vi "RequestFIFO.vi"   [LabVIEW 2018]
uses:
  <vilib>/rvi/Emulation/niFpgaGetClockAttributes.vi
  <vilib>/rvi/Emulation/niFpgaSctlEmulationGetInTimedLoop.vi
  <vilib>/rvi/Emulation/niFpgaEmulationReportErrorSimple.vi
  <vilib>/rvi/interface/RandomDataEmulation/niFpgaRandomDataHandleErrors.vi
  <vilib>/rvi/Emulation/niFpgaEmulationIsFPGAContextNoSignature.vi
  <vilib>/rvi/errors/niFpgaSetErrorForExecOnDevCompSimple.vi
  <vilib>/rvi/eio/common/nirviEmuReportErrorAndStop.vi
  <vilib>/rvi/DataTransferAndStorage/Container/Common/niFpgaContainerGetUniqueNameForEmu.vi
  <vilib>/rvi/FIFO/Fifo_Resource/nirvififoEmulationSetSize.vi
  <vilib>/rvi/FIFO/Fifo_Resource/nirviFifoEmulationQueueMgr.vi
  <instcachedir>/0/nirviFifoEmulationQueueMgr_E5CAEC123FF24DC58D834DCA3CDAA9B5.lvgen/nirviFifoEmulationQueueMgr_E5CAEC123FF24DC58D834DCA3CDAA9B5_032.vi
  <vilib>/Utility/error.llb/Clear Errors.vi
  <vilib>/rvi/FIFO/Fifo_Resource/nirvififoEmulationCreateLock.vi
  <vilib>/rvi/Emulation/niFpgaProcessEmulError.vi
  <vilib>/rvi/FIFO/Fifo_Resource/nirvififoEmulationObtainLock.vi
  <vilib>/rvi/FIFO/Fifo_Resource/nirvififoEmulationReleaseLock.vi
  <vilib>/rvi/occurrence/nirviWaitOnOccurrenceBase.vi
  <vilib>/rvi/errors/nirviReportUnexpectedCaseInternalError.vi
  <vilib>/rvi/errors/nirviReportUnexpectedCaseInternalError (U32).vi
  <vilib>/rvi/eio/common/nirviEmuTemplateMethod_errors.vi
  <vilib>/rvi/Emulation/niFpgaCriticalErrorInLSC.vi
  <vilib>/rvi/DataTransferAndStorage/Container/XNode/niFpgaContainer.xnode
  <vilib>/rvi/interface/RandomDataEmulation/nirviRandomDataFpgaReadWriteTemplate.vi
  <vilib>/rvi/FIFO/Fifo_Resource/nirvififoEmulationRead.vi
  <vilib>/eio/EIONode/EIONode.xnode
types:
  T1 = typedef "Addresses.ctl" = enum8{"NA", "Accelerometers", "Timestamp", "ChasisTemperature"}
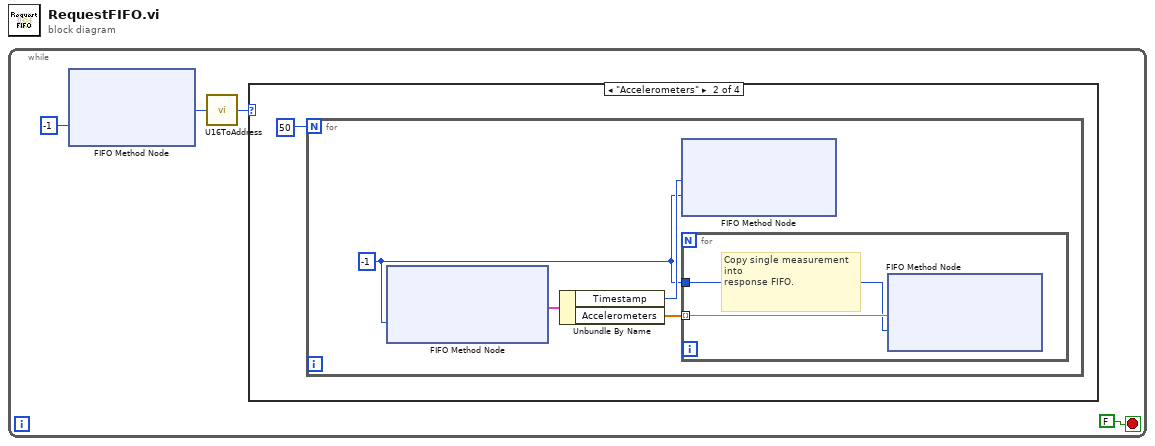
[diagram p0: block diagram]
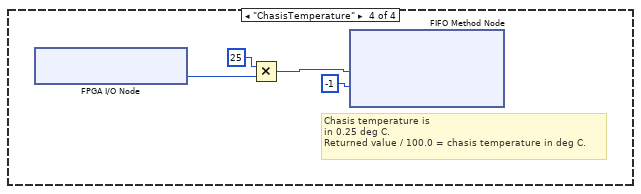
[diagram p4: hidden frame]
diagram:
  n1 = while {
    stop <- FALSE stop-if-true
    n2 = xnode ("FIFO Method Node")("Timeout"=-1) -> ("Element"=w2:u16)  [unwired: 1 in, 2 out]
    n3 = call "U16ToAddress.vi"("Input"=w2) -> ("Addresses"=w1:T1)
    n4 = case shown="\"Accelerometers\"" w1 {
      frame "NA" {
      }
      frame "Accelerometers" {
        n5 = for {
          N: 50 -> [_]
          w6 = -1 ("Timeout")
          n6 = xnode ("FIFO Method Node")("Timeout"=w6) -> ("Element"=w9:cluster{"Timestamp":u64, "Accelerometers":sgl[]})  [unwired: 1 in, 2 out]
          n7 = Unbundle By Name(w9) -> ("Timestamp"=w8:u64, "Accelerometers"=w7:sgl[])
          n8 = xnode ("FIFO Method Node")("Element"=w8, "Timeout"=w6) -> ()  [unwired: 1 in, 2 out]
          n9 = for {
            tunnel: w7 -> [w11] mode=indexing
            tunnel: w6 -> [w10]
            # "Copy single measurement into\nresponse FIFO."
            n10 = xnode ("FIFO Method Node")("Element"=w11, "Timeout"=w10) -> ()  [unwired: 1 in, 2 out]
          }
        }
      }
      frame "Timestamp" {
      }
      frame "ChasisTemperature" {
        # "Chasis temperature is\nin 0.25 deg C.\nReturned value / 100.0 = chasis temperature in deg C."
        n11 = xnode "FPGA I/O Node"() -> ("Chassis Temperature"=w14:i16)  [unwired: 1 in, 1 out]
        n12 = Multiply(x=i16 25, y=w14) -> (x*y=w12:i16)
        n13 = xnode ("FIFO Method Node")("Element"=w12, "Timeout"=-1) -> ()  [unwired: 1 in, 2 out]
      }
    }
  }
